vi "Parse XML for Tags.vi"(8 "error in (no error)":errorcluster, 10 "xml string":string) -> (0 "error out":errorcluster, 3 "xml structure":T1)   [LabVIEW 2013]
uses:
  XML Structure - Cluster.ctl
  XML Tag Type - Enum.ctl
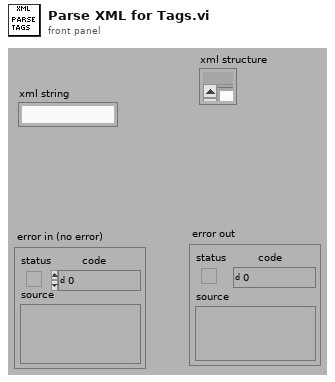
[diagram p1: front panel]
types:
  T1 = typedef "XML Structure - Cluster.ctl" = cluster{"tags":string[], "tag names":string[], "tag type":T2[], "offset":i32[], "close tag index":i32[], "xml":string, "Children":cluster{"children":i32[]}[], "parent index":i32[]}
  T2 = typedef "XML Tag Type - Enum.ctl" = enum16{"start tag", "empty tag", "end tag"}
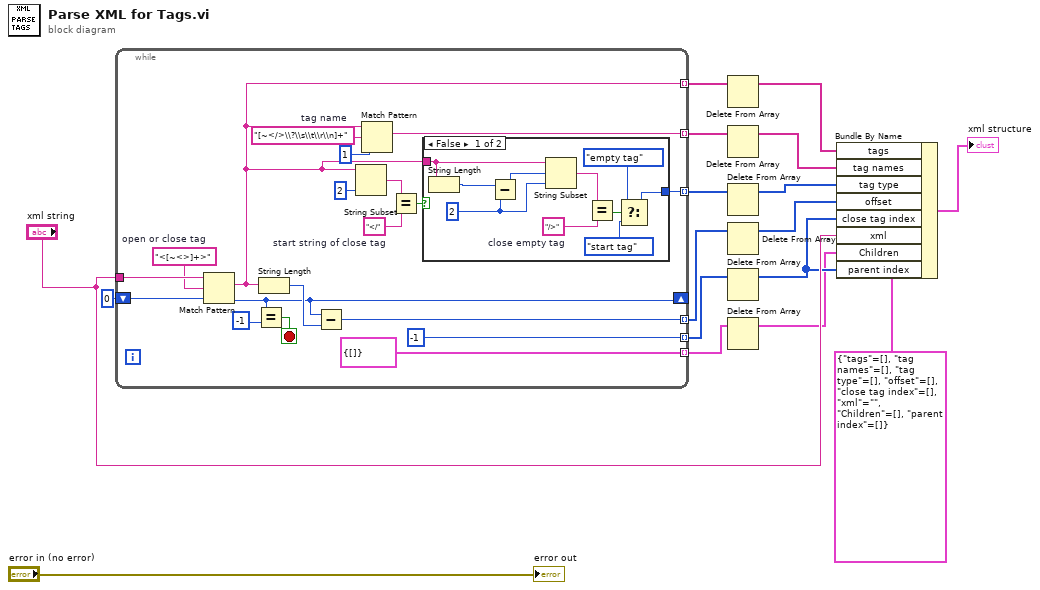
[diagram p0: block diagram]
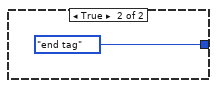
[diagram p2: hidden frame]
diagram:
  n1 = while {
    tunnel: "xml string" -> [w36]
    shift-right: [w24] -> _
    shift-left: 0 ("offset past match") -> [w35]
    tunnel: [w18] -> w15 mode=indexing
    tunnel: [w19] -> w16 mode=indexing
    tunnel: [w26] -> w17 mode=indexing
    tunnel: [w23] -> w5 mode=indexing
    tunnel: [-1 ("offset past match")] -> w3 mode=indexing
    tunnel: [cluster{"children":i32[]} {"children"=[]} ("Children")] -> w1 mode=indexing
    stop <- w32 stop-if-true
    w31 = "[~</>\\?\\s\\t\\r\\n]+"  # tag name
    w27 = "</"  # start string of close tag
    w34 = "<[~<>]+>"  # open or close tag
    n2 = Match Pattern(string=w36, regular expression=w34, offset (0)=w35) -> (match substring=w18:string, offset past match=w24:i32)  [unwired: 2 out]
    n3 = Equal?(x=w24, y=-1 ("offset past match")) -> (x = y?=w32:bool)
    n4 = String Length(string=w18) -> (length=w25:i32)
    n5 = Subtract(x=w24, y=w25) -> (x-y=w23:i32)
    n6 = String Subset(string=w18, length (rest)=2 ("length (rest)")) -> (substring=w28:string)  [unwired: 1 in]
    n7 = Match Pattern(string=w18, regular expression=w31, offset (0)=1) -> (match substring=w26:string)  [unwired: 3 out]
    n8 = Equal?(x=w28, y=w27) -> (x = y?=w20:bool)
    n9 = case shown="False" w20 {
      tunnel: [w38 XML_Tag_Type_-_Enum."end tag" ("tag type")] -> w19
      tunnel: w18 -> [w46 _]
      frame False {
        w42 = "/>"  # close empty tag
        w45 = 2 ("length (rest)")
        n10 = String Length(string=w46) -> (length=w37:i32)
        n11 = Subtract(x=w37, y=w45) -> (x-y=w44:i32)
        n12 = String Subset(string=w46, offset (0)=w44, length (rest)=w45) -> (substring=w43:string)
        n13 = Equal?(x=w43, y=w42) -> (x = y?=w41:bool)
        n14 = Select(t=XML_Tag_Type_-_Enum."empty tag" ("tag type"), s=w41, f=XML_Tag_Type_-_Enum."start tag" ("tag type")) -> (s? t:f=w38:T2)
      }
      frame True {
      }
    }
  }
  n15 = Delete From Array(array=w15) -> (array with subset deleted=w12:string[])  [unwired: 2 in, 1 out]
  n16 = Delete From Array(array=w17) -> (array with subset deleted=w11:string[])  [unwired: 2 in, 1 out]
  n17 = Delete From Array(array=w16) -> (array with subset deleted=w10:T2[])  [unwired: 2 in, 1 out]
  n18 = Delete From Array(array=w5) -> (array with subset deleted=w6:i32[])  [unwired: 2 in, 1 out]
  n19 = Delete From Array(array=w3) -> (array with subset deleted=w4:i32[])  [unwired: 2 in, 1 out]
  n20 = Delete From Array(array=w1) -> (array with subset deleted=w2:cluster{"children":i32[]}[])  [unwired: 2 in, 1 out]
  n21 = Bundle By Name(cluster=T1 {"tags"=[], "tag names"=[], "tag type"=[], "offset"=[], "close tag index"=[], "xml"="", "Children"=[], "parent index"=[]} ("xml structure"), "tags"=w12, "tag names"=w11, "tag type"=w10, "offset"=w6, "close tag index"=w4, "xml"="xml string", "Children"=w2, "parent index"=w4) -> (→"xml structure":T1)
  "error out" <- "error in (no error)"
